vi "Open Build.vi"(8 "error in (no error)":errorcluster, 10 "Build specification name":string, 11 "TargetItem Refnum":refnum<vi>) -> (0 "error out":errorcluster, 3 "DSDIST out":refnum<class "NI_AB_API_DSDIST.lvclass">)   [LabVIEW 2020, in "NI_AB_API_DSDIST.lvclass"]
uses:
  <vilib>/AppBuilder/AB_API/DSDIST/NI_AB_API_DSDIST.lvclass
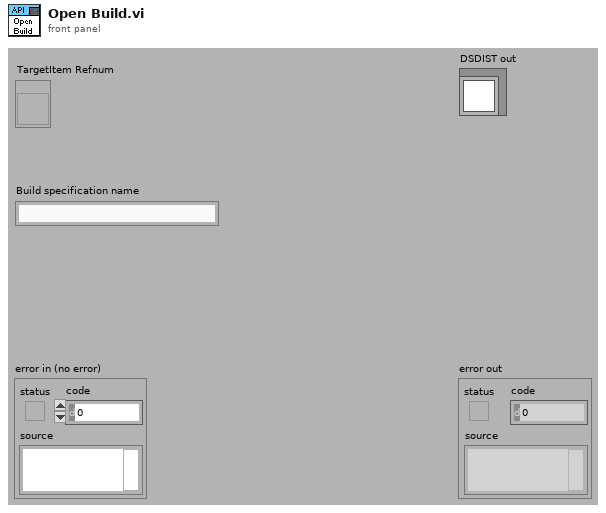
[diagram p1: front panel]
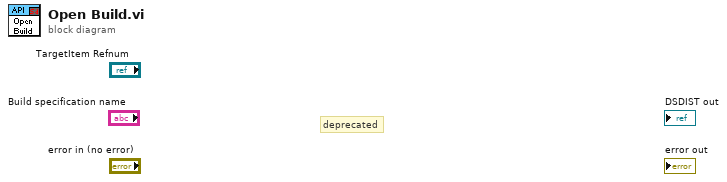
[diagram p0: block diagram]
diagram:
  # "deprecated"
